vi "DetermineChangeToTimingIncrementButtons.vi"() -> (1 "Increment":string, 2 "Position":cluster{"Card":dbl, "Channel":dbl})   [LabVIEW 2013]
doc: "Determines the change to the timing cluster that generated the event and prepares a job.\n\nThe change in the timing cluster is determined by comparing old and new values of each elment fo the timing cluster. It is assumed that only one value can change per event. i.e. the computer can process events faster than the user can generate them. \nThe VI prepares a job for the consumer loop to do with information on where the change occured."
uses:
  Controls/TimingArrayEventJob.ctl
  Controls/TimeIncrementCluster.ctl
panel:
  in  "TimingIncrement New":T1
  in  "TimingIncrement Old":T1
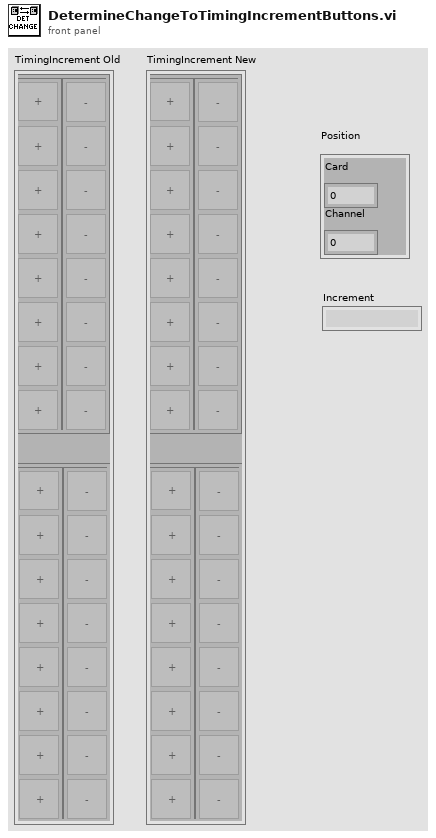
[diagram p1: front panel]
types:
  T1 = typedef "TimeIncrementCluster.ctl" = cluster{"Plus Minus":cluster{"Add 1":cluster{"plus 1":bool, "plus 2":bool, "plus 3":bool, "plus 4":bool, "plus 5":bool, "plus 6":bool, "plus 7":bool, "plus 8":bool}, "Minus 1":cluster{"minus 1":bool, "minus 2":bool, "minus 3":bool, "minus 4":bool, "minus 5":bool, "minus 6":bool, "minus 7":bool, "minus 8":bool}}, "Plus Minus 2":cluster{"Add 1":cluster{"plus 1":bool, "plus 2":bool, "plus 3":bool, "plus 4":bool, "plus 5":bool, "plus 6":bool, "plus 7":bool, "plus 8":bool}, "Minus 1":cluster{"minus 1":bool, "minus 2":bool, "minus 3":bool, "minus 4":bool, "minus 5":bool, "minus 6":bool, "minus 7":bool, "minus 8":bool}}}
  T2 = typedef "TimingArrayEventJob.ctl" = enum16{"Enable/Dis", "Redraw Timing Plot", "Do Nothing"}
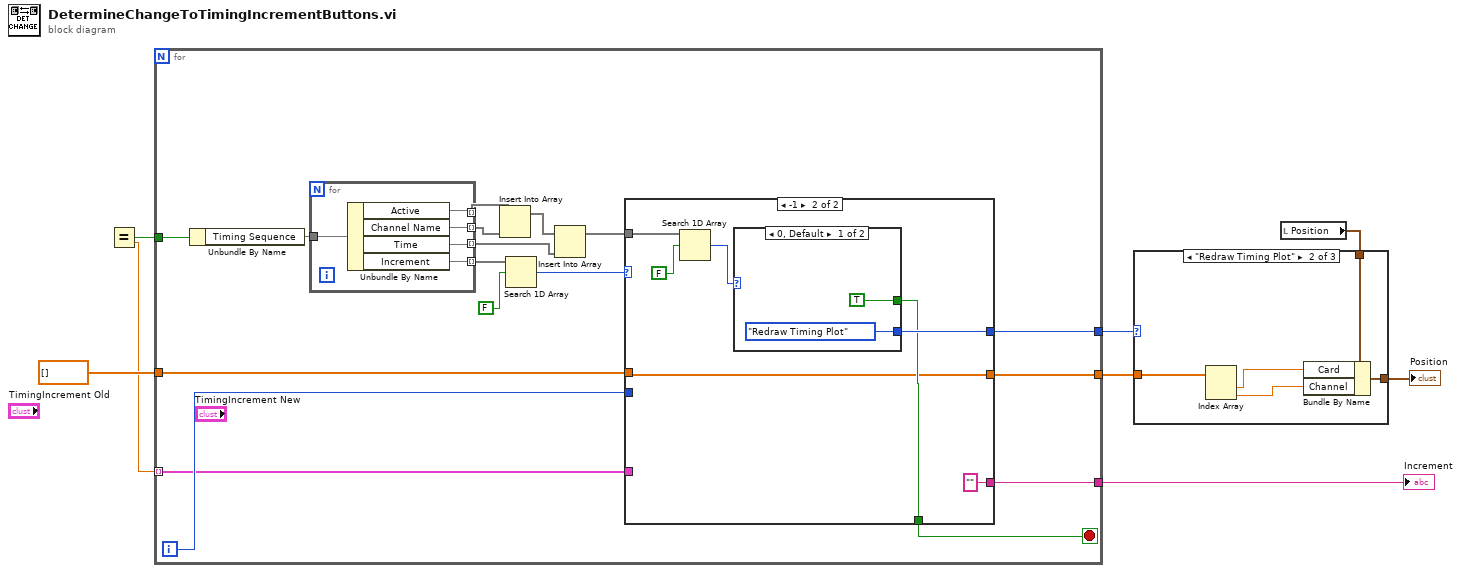
[diagram p0: block diagram]
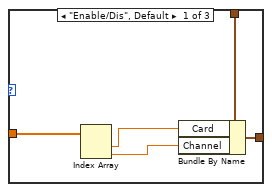
[diagram p2: hidden frame]
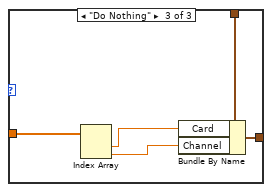
[diagram p3: hidden frame]
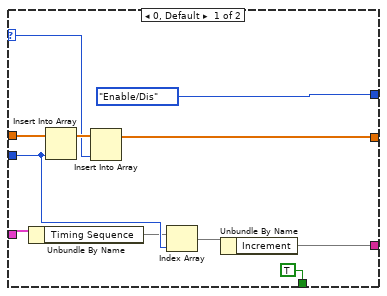
[diagram p4: hidden frame]
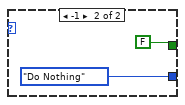
[diagram p5: hidden frame]
diagram:
  n1 = Equal?() -> (x=w9:dbl, y=w2:dbl, x = y?=w8:bool)
  n2 = for {
    tunnel: w8 -> [w12]
    tunnel: [w26] -> w3
    tunnel: [w25] -> w6
    tunnel: dbl[] [] ("Location") -> [w24]
    tunnel: w2 -> [w11] mode=indexing
    tunnel: [w10] -> w1
    i -> [w23]
    stop <- w22 stop-if-true
    n3 = Unbundle By Name(w12) -> ("Timing Sequence"=w21)
    n4 = for {
      tunnel: w21 -> [w53]
      tunnel: [w52] -> w17 mode=indexing
      tunnel: [w51] -> w16 mode=indexing
      tunnel: [w50] -> w14 mode=indexing
      tunnel: [w49] -> w20 mode=indexing
      n5 = Unbundle By Name(w53) -> ("Active"=w52, "Channel Name"=w51, "Time"=w50, "Increment"=w49)
    }
    n6 = Insert Into Array(array=w17, new element=w16) -> (w15:void[])  [unwired: 1 in]
    n7 = Search 1D Array(1D array=w20, element=FALSE) -> (index of element=w18:i32)  [unwired: 1 in]
    n8 = Insert Into Array(array=w15, new element=w14) -> (w13:void[])  [unwired: 1 in]
    n9 = case shown="-1" w18 {
      selector: w18 -> [w30 _]
      tunnel: w13 -> [_ w44]
      tunnel: [TimingArrayEventJob."Enable/Dis" ("Job") w41] -> w26
      tunnel: [w34 w39] -> w25
      tunnel: w24 -> [w36 w39]
      tunnel: w23 -> [w31 _]
      tunnel: [TRUE w40] -> w22
      tunnel: w11 -> [w32 _]
      tunnel: [w27 "" ("Increment")] -> w10
      frame 0, Default {
        n10 = Unbundle By Name(w32) -> ("Timing Sequence"=w29)
        n11 = Insert Into Array(array=w36, new element=w31) -> (w35:dbl[])  [unwired: 1 in]
        n12 = Insert Into Array(array=w35, new element=w30) -> (w34:dbl[])  [unwired: 1 in]
        n13 = Index Array(array=w29, index=w31) -> (element=w28)
        n14 = Unbundle By Name(w28) -> ("Increment"=w27)
      }
      frame -1 {
        n15 = Search 1D Array(1D array=w44, element=FALSE) -> (index of element=w42:i32)  [unwired: 1 in]
        n16 = case shown="0, Default" w42 {
          tunnel: [TimingArrayEventJob."Redraw Timing Plot" ("Job") TimingArrayEventJob."Do Nothing" ("Job")] -> w41
          tunnel: [TRUE FALSE] -> w40
          frame 0, Default {
          }
          frame -1 {
          }
        }
      }
    }
  }
  "Increment" <- w1
  n17 = local read "Position"() -> (w5:cluster{"Card":dbl, "Channel":dbl})
  n18 = case shown="\"Redraw Timing Plot\"" w3 {
    tunnel: w6 -> [w58 w63 w68]
    tunnel: w5 -> [w57 w62 w67]
    tunnel: [w54 w59 w64] -> w4
    frame "Enable/Dis", Default {
      n19 = Index Array(array=w58) -> (element #1=w56:dbl, element #2=w55:dbl)  [unwired: 2 in]
      n20 = Bundle By Name(cluster=w57, "Card"=w56, "Channel"=w55) -> (w54:cluster{"Card":dbl, "Channel":dbl})
    }
    frame "Redraw Timing Plot" {
      n21 = Index Array(array=w63) -> (element #1=w61:dbl, element #2=w60:dbl)  [unwired: 2 in]
      n22 = Bundle By Name(cluster=w62, "Card"=w61, "Channel"=w60) -> (w59:cluster{"Card":dbl, "Channel":dbl})
    }
    frame "Do Nothing" {
      n23 = Index Array(array=w68) -> (element #1=w66:dbl, element #2=w65:dbl)  [unwired: 2 in]
      n24 = Bundle By Name(cluster=w67, "Card"=w66, "Channel"=w65) -> (w64:cluster{"Card":dbl, "Channel":dbl})
    }
  }
  "Position" <- w4
